vi "Initialization VI.vi"(8 "error in (no error)":errorcluster, 10 "Custom XML":string, 11 "Device Item Ref in":T1 format="%.0x") -> (0 "error out":errorcluster, 3 "Device Item Ref out":T1 format="%.0x")   [LabVIEW 2019, in "OPC UA Client Addon System Explorer.lvlib"]
uses:
  OPC UA Client Addon System Explorer.lvlib
  <vilib>/NI VeriStand/Custom Device API/Custom Device Item Ref.ctl
  <vilib>/NI VeriStand/Custom Device API/Custom Device Channel.ctl
  <vilib>/NI VeriStand/Custom Device API/Custom Device Channel Type.ctl
  Addon Shared/SubVIs/Constants.vi
  <vilib>/NI VeriStand/Custom Device API/Custom Device API.lvlib
  Addon Shared/OPC UA Client Addon Shared.lvlib
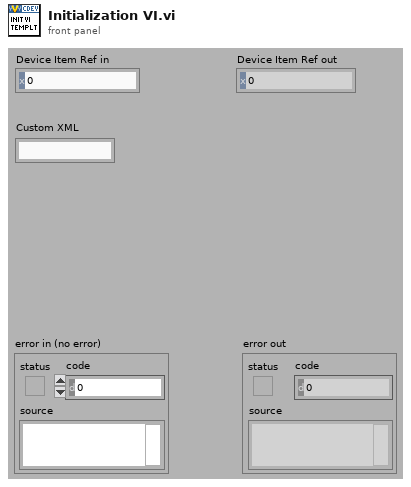
[diagram p1: front panel]
types:
  T1 = typedef "Custom Device API.lvlib/Custom Device Item Ref.ctl" = u64
  T2 = typedef "Custom Device API.lvlib/Custom Device Channel.ctl" = cluster{"Type":T3, "Units":string, "Default Value":dbl, "Faultable":bool, "Scalable":bool}
  T3 = typedef "Custom Device API.lvlib/Custom Device Channel Type.ctl" = enum16{"Input", "Output"}
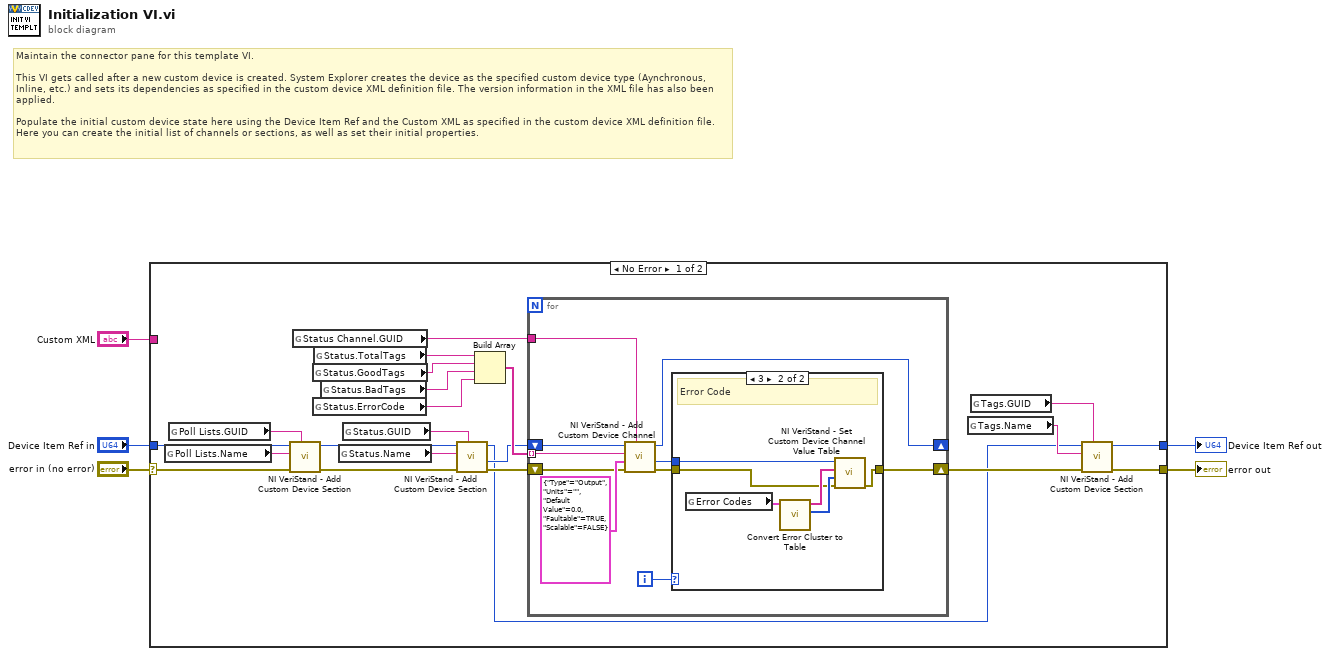
[diagram p0: block diagram]
diagram:
  # "Maintain the connector pane for this template VI.\n\nThis VI gets called after a new custom device is created. System Explorer creates the device as the specified custom device type (Aynchronous, Inline, etc.) and sets its dependencies as specified in the custom device XML definition file. The version information in the XML file has also been applied.\n\nPopulate the initial custom device state here using the Device Item Ref and the Custom XML as specified in the custom device XML definition file. Here you can create the initial list of channels or sections, as well as set their initial properties."
  n1 = case shown="No Error" "error in (no error)" {
    selector: "error in (no error)" -> [w19 w46]
    tunnel: [w25 w46] -> w5
    tunnel: [w24 w45] -> w3
    tunnel: "Device Item Ref in" -> [w17 w45]
    tunnel: "Custom XML" -> [_ _]
    frame No Error {
      n2 = global read "Constants.vi" "Poll Lists.Name"() -> (w21:string)
      n3 = global read "Constants.vi" "Poll Lists.GUID"() -> (w20:string)
      n4 = call <vilib>:"NI VeriStand - Add Custom Device Section.vi"("GUID (Default Section)"=w20, "error in (no error)"=w19, "Section Name"=w21, "Parent Ref in"=w17) -> ("error out"=w18:errorcluster, "Parent Ref out"=w16:T1)  [unwired: 4 in, 2 out]
      n5 = global read "Constants.vi" "Status Channel.GUID"() -> (w9:string)
      n6 = global read "Constants.vi" "Status.GoodTags"() -> (w14:string)
      n7 = global read "Constants.vi" "Status.ErrorCode"() -> (w6:string)
      n8 = global read "Constants.vi" "Status.TotalTags"() -> (w15:string)
      n9 = global read "Constants.vi" "Status.BadTags"() -> (w13:string)
      n10 = global read "Constants.vi" "Status.Name"() -> (w26:string)
      n11 = global read "Constants.vi" "Status.GUID"() -> (w27:string)
      n12 = call <vilib>:"NI VeriStand - Add Custom Device Section.vi"("GUID (Default Section)"=w27, "error in (no error)"=w18, "Section Name"=w26, "Parent Ref in"=w16) -> ("error out"=w12:errorcluster, "Section Ptr"=w8:T1, "Parent Ref out"=w7:T1)  [unwired: 4 in, 1 out]
      n13 = Build Array(w15, w14, w13, w6) -> (w10:string[])
      n14 = for {
        shift-right: [w35] -> _
        shift-left: w8 -> [w36]
        shift-right: [w28] -> w11
        shift-left: w12 -> [w34]
        tunnel: w10 -> [w33] mode=indexing
        tunnel: w9 -> [w32]
        i -> [w31]
        n15 = call <vilib>:"NI VeriStand - Add Custom Device Channel.vi"("GUID (Default Channel)"=w32, "error in (no error)"=w34, "Channel"=T2 {"Type"=enum."Output", "Units"="", "Default Value"=0.0, "Faultable"=TRUE, "Scalable"=FALSE}, "Channel Name"=w33, "Parent Ref in"=w36) -> ("error out"=w29:errorcluster, "Channel Ref"=w30:T1, "Parent Ref out"=w35:T1)  [unwired: 3 in, 1 out]
        n16 = case shown="3" w31 {
          tunnel: w30 -> [_ w41]
          tunnel: w29 -> [w38 w40]
          tunnel: [w38 w39] -> w28
          frame 0, Default {
          }
          frame 3 {
            # "Error Code"
            n17 = global read "Constants.vi" "Error Codes"() -> (w42:cluster{"number":i32, "trimmed string":string}[])
            n18 = call "Convert Error Cluster to Table.vi"("Error Codes"=w42) -> ("Code"=w43:i32[], "String"=w44:string[])  [unwired: 9 in]
            n19 = call <vilib>:"NI VeriStand - Set Custom Device Channel Value Table.vi"("error in (no error)"=w40, "Values"=w43, "Names"=w44, "Channel Ref in"=w41) -> ("error out"=w39:errorcluster)  [unwired: 6 in, 1 out]
          }
        }
      }
      n20 = global read "Constants.vi" "Tags.Name"() -> (w22:string)
      n21 = global read "Constants.vi" "Tags.GUID"() -> (w23:string)
      n22 = call <vilib>:"NI VeriStand - Add Custom Device Section.vi"("GUID (Default Section)"=w23, "error in (no error)"=w11, "Section Name"=w22, "Parent Ref in"=w7) -> ("error out"=w25:errorcluster, "Parent Ref out"=w24:T1)  [unwired: 4 in, 2 out]
    }
    frame Error {
    }
  }
  "error out" <- w5
  "Device Item Ref out" <- w3
